vi "Key Sequence JSON.vi"(11 "Key Sequence":T1) -> (3 "Key Sequence JSON":string)   [LabVIEW 2022 SP3, in "obs-websocket-lv.lvlib"]
uses:
  obs-websocket-lv.lvlib
  Key Sequence.ctl
  OBS Key.ctl
  <vilib>/IlluminatedG/lv-web-crypto/lv-json/JSON/JSON.lvlib
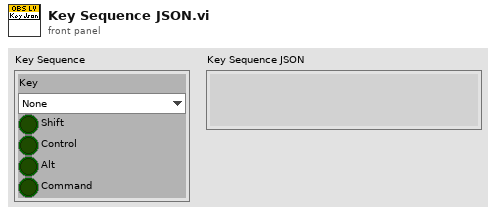
[diagram p1: front panel]
types:
  T1 = typedef "obs-websocket-lv.lvlib/Key Sequence.ctl" = cluster{"Key":T2, "Shift":bool, "Control":bool, "Alt":bool, "Command":bool}
  T2 = typedef "obs-websocket-lv.lvlib/OBS Key.ctl" = enum16{"None", "Return", "Enter", "Escape", "Tab", "Backtab", "Backspace", "Insert", "Delete", "Pause", "Print", "SysReq", "Clear", "Home", "End", "Left", "Up", "Right", "Down", "PageUp", "PageDown", "Shift", "Control", "Meta", "Alt", "AltGr", "Capslock", "Numlock", "Scrolllock", "F1", "F2", "F3", "F4", "F5", "F6", "F7", "F8", "F9", "F10", "F11", "F12", "F13", "F14", "F15", "F16", "F17", "F18", "F19", "F20", "F21", "F22", "F23", "F24", "F25", "F26", "F27", "F28", "F29", "F30", "F31", "F32", "F33", "F34", "F35", "Menu", "Hyper_L", "Hyper_R", "Help", "Direction_L", "Direction_R", "Space", "Exclam", "QuoteDbl", "NumberSign", "Dollar", "Percent", "Ampersand", "Apostrophe", "ParenLeft", "ParenRight", "Asterisk", "Plus", "Comma", "Minus", "Period", "Slash", "0", "1", "2", "3", "4", "5", "6", "7", "8", "9", "NumEqual", "NumAsterisk", "NumPlus", "NumComma", "NumMinus", "NumPeriod", "NumSlash", "Num0", "Num1", "Num2", "Num3", "Num4", "Num5", "Num6", "Num7", "Num8", "Num9", "Colon", "Semicolon", "Quote", "Less", "Equal", "Greater", "Question", "At", "A", "B", "C", "D", "E", "F", "G", "H", "I", "J", "K", "L", "M", "N", "O", "P", "Q", "R", "S", "T", "U", "V", "W", "X", "Y", "Z", "BracketLeft", "Backslash", "BracketRight", "AsciiCircum", "Underscore", "QuoteLeft", "BraceLeft", "Bar", "BraceRight", "AsciiTilde", "NoBreakSpace", "ExclamDown", "Cent", "Sterling", "Currency", "Yen", "Brokenbar", "Section", "Diaresis", "Copyright", "OrdFeminine", "GuillemotLeft", "NotSign", "Hyphen", "Registered", "Macron", "Degree", "PlusMinus", "TwoSuperior", "ThreeSuperior", "Acute", "Mu", "Paragraph", "PeriodCentered", "Cedilla", "OneSuperior", "Masculine", "GuillemotRight", "OneQuarter", "OneHalf", "ThreeQuarters", "QuestionDown", "Agrave", "AAcute", "ACircumflex", "ATilde", "ADiaresis", "ARing", "AE", "CCedilla", "EGrave", "EAcute", "ECircumflex", "EDiaresis", "IGrave", "IAcute", "ICircumflex", "IDiaresis", "Eth", "NTilde", "OGrave", "OAcute", "OCircumflex", "OTilde", "ODiaresis", "Multiply", "OOblique", "UGrave", "UAcute", "UCircumflex", "UDiaresis", "YAcute", "Thorn", "SSharp", "Division", "YDiaresis", "Multi_Key", "CodeInput", "SingleCandidate", "MultipleCandidate", "PreviousCandidate", "Mode_Switch", "Kanji", "Muhenkan", "Henkan", "Romaji", "Hiragana", "Katakana", "Hiragana_Katakana", "Zenkaku", "Hankaku", "Zenkaku_Hankaku", "Touroku", "Massyo", "Kana_Lock", "Kana_Shift", "Eisu_Shift", "Eisu_Toggle", "Hangul", "Hangul_Start", "Hangul_End", "Hangul_Hanja", "Hangul_Jamo", "Hangul_Romaja", "Hangul_Jeonja", "Hangul_Banja", "Hangul_Prehanja", "Hangul_Posthanja", "Hangul_Special", "Dead_Grave", "Dead_Acute", "Dead_Circumflex", "Dead_Tilde", "Dead_Macron", "Dead_Breve", "Dead_AboveDot", "Dead_Diaresis", "Dead_AboveRing", "Dead_DoubleAcute", "Dead_Caron", "Dead_Cedilla", "Dead_Ogonek", "Dead_Iota", "Dead_Voiced_Sound", "Dead_Semivoiced_Sound", "Dead_BelowDot", "Dead_Hook", "Dead_Horn", "Back", "Forward", "Stop", "Refresh", "VolumeDown", "VolumeMute", "VolumeUp", "BassBoost", "BassUp", "BassDown", "TrebleUp", "TrebleDown", "MediaPlay", "MediaStop", "MediaPrevious", "MediaNext", "MediaRecord", "MediaPause", "MediaTogglePlayPause", "Homepage", "Favorites", "Search", "Standby", "OpenURL", "LaunchMail", "LaunchMedia", "Launch0", "Launch1", "Launch2", "Launch3", "Launch4", "Launch5", "Launch6", "Launch7", "Launch8", "Launch9", "LaunchA", "LaunchB", "LaunchC", "LaunchD", "LaunchE", "LaunchF", "LaunchG", "LaunchH", "MonBrightnessUp", "MonBrightnessDown", "KeyboardLightOnOff", "KeyboardBrightnessUp", "KeyboardBrightnessDown", "Poweroff", "Wakeup", "Eject", "Screensaver", "WWW", "Memo", "Lightbulb", "Shop", "History", "AddFavorite", "Hotlinks", "BrightnessAdjust", "Finance", "Community", "AudioRewind", "BackForward", "ApplicationLeft", "ApplicationRight", "Book", "CD", "Calculator", "TodoList", "ClearGrab", "Close", "Copy", "Cut", "Display", "DOS", "Documents", "Excel", "Explorer", "Game", "Go", "ITouch", "Logoff", "Market", "Meeting", "MenuKB", "MenuPB", "MySites", "News", "OfficeHome", "Option", "Paste", "Phone", "Calendar", "Reply", "Reload", "RotateWindows", "RotationPB", "RotationKB", "Save", "Send", "Spell", "SplitScreen", "Support", "TakePane", "Terminal", "Tools", "Travel", "Video", "Word", "Xfer", "ZoomIn", "ZoomOut", "Away", "Messenger", "Webcam", "MailForward", "Pictures", "Music", "Battery", "Bluetooth", "WLan", "UWB", "AudioForward", "AudioRepeat", "AudioRandomPlay", "Subtitle", "AudioCycleTrack", "Time", "Hibernate", "View", "TopMenu", "Powerdown", "Suspend", "ContrastAdjust", "MediaLast", "Call", "Camera", "CameraFocus", "Context1", "Context2", "Context3", "Context4", "Flip", "Hangup", "No", "Select", "Yes", "ToggleCallHangup", "VoiceDial", "LastNumberRedial", "Execute", "Printer", "Play", "Sleep", "Zoom", "Cancel", "Mouse1", "Mouse2", "Mouse3", "Mouse4", "Mouse5", "Mouse6", "Mouse7", "Mouse8", "Mouse9", "Mouse10", "Mouse11", "Mouse12", "Mouse13", "Mouse14", "Mouse15", "Mouse16", "Mouse17", "Mouse18", "Mouse19", "Mouse20", "Mouse21", "Mouse22", "Mouse23", "Mouse24", "Mouse25", "Mouse26", "Mouse27", "Mouse28", "Mouse29", "Backslash_RT102", "Open", "Find", "Redo", "Undo", "Front", "Props"}
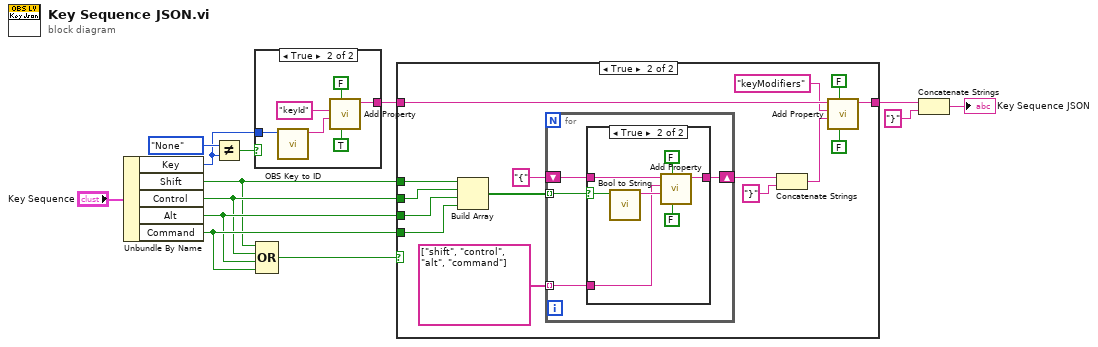
[diagram p0: block diagram]
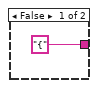
[diagram p4: hidden frame]
diagram:
  n1 = Unbundle By Name("Key Sequence") -> ("Key"=w10:T2, "Shift"=w5:bool, "Control"=w6:bool, "Alt"=w7:bool, "Command"=w8:bool)
  n2 = Not Equal?(x=OBS_Key."None", y=w10) -> (x != y?=w11:bool)
  n3 = case shown="True" w11 {
    tunnel: w10 -> [_ w17]
    tunnel: ["{" ("String out") w15] -> w4
    frame False {
    }
    frame True {
      n4 = call "OBS Key to ID.vi"("OBS Key"=w17) -> ("Key ID"=w16:string)  [unwired: 10 in]
      n5 = call <vilib>:"Add Property.vi"("String?"=TRUE, "Include Empty?"=FALSE, "Value"=w16, "Property Name"="keyId") -> ("String out"=w15:string)  [unwired: 7 in]
    }
  }
  n6 = Compound Arithmetic op=OR(w5, w6, w7, w8) -> (w9:bool)
  n7 = case shown="True" w9 {
    tunnel: w8 -> [_ w33]
    tunnel: w7 -> [_ w34]
    tunnel: w6 -> [_ w35]
    tunnel: w5 -> [_ w36]
    tunnel: w4 -> [w21 w27]
    tunnel: [w21 w24] -> w3
    frame False {
    }
    frame True {
      n8 = Build Array(w36, w35, w34, w33) -> (w32:bool[])
      n9 = for {
        tunnel: w32 -> [w39] mode=indexing
        shift-right: [w37] -> w29
        shift-left: "{" -> [w40]
        tunnel: string[] ["shift", "control", "alt", "command"] -> [w38] mode=indexing
        n10 = case shown="True" w39 {
          selector: w39 -> [_ w48]
          tunnel: w40 -> [w41 w47]
          tunnel: w38 -> [_ w45]
          tunnel: [w41 w44] -> w37
          frame False {
          }
          frame True {
            n11 = call <vilib>:"Bool to String.vi"("Boolean"=w48) -> ("Value"=w46:string)  [unwired: 10 in]
            n12 = call <vilib>:"Add Property.vi"("String?"=FALSE, "Include Empty?"=FALSE ("String?"), "Value"=w46, "Property Name"=w45, "String In"=w47) -> ("String out"=w44:string)  [unwired: 6 in]
          }
        }
      }
      n13 = Concatenate Strings(w29, "}" ("string")) -> (w26:string)
      n14 = call <vilib>:"Add Property.vi"("String?"=FALSE, "Include Empty?"=FALSE ("String?"), "Value"=w26, "Property Name"="keyModifiers", "String In"=w27) -> ("String out"=w24:string)  [unwired: 6 in]
    }
  }
  n15 = Concatenate Strings(w3, "}" ("string")) -> (→"Key Sequence JSON":string)
